vi "api_demo.vi"() -> ()   [LabVIEW 2017]
panel:
  in  "地址":string="127.0.0.1"
  in  "刷新":bool
  out "cz":dbl
  out "cy":dbl
  out "cx":dbl
  in  "LET":enum32{"回零", "扫描", "手动", "配置"}(tab)
  in  "组合框":string(combo)
  in  "去，并设置原点":bool
  in  "运行速度":dbl=50.0
  in  "去":bool
  in  "目标z":dbl
  in  "目标y":dbl=100.0
  in  "目标x":dbl=100.0
  in  "回零速度":dbl=20.0
  in  "回零":bool
  in  "slopey":dbl=100.0
  in  "slopex":dbl=100.0
  in  "ydir":bool=TRUE
  in  "xdir":bool=TRUE
  in  "scan v":dbl=50.0
  in  "退出扫描":bool
  in  "下一步":bool
  in  "开始":bool
  in  "type":string(combo)="zigzagx"
  out "状态":string
  in  "speed":dbl=50.0
  in  "step":dbl=50.0
  in  "Z-":bool
  in  "Z+":bool
  in  "Y+":bool
  in  "Y-":bool
  in  "X-":bool
  in  "X+":bool
  in  "复位":bool
  in  "刷新数值":bool
  in  "configrv":bool
  in  "configgap":bool
  in  "configwhz":bool
  in  "configdxdy":bool
  in  "configoxyz":bool
  in  "rv":dbl
  in  "zhome":dbl
  in  "gapspeed":dbl
  in  "gap":dbl
  in  "d":dbl
  in  "w":dbl
  in  "h":dbl
  in  "d2":dbl
  in  "d1":dbl
  in  "oz":dbl
  in  "oy":dbl
  in  "ox":dbl
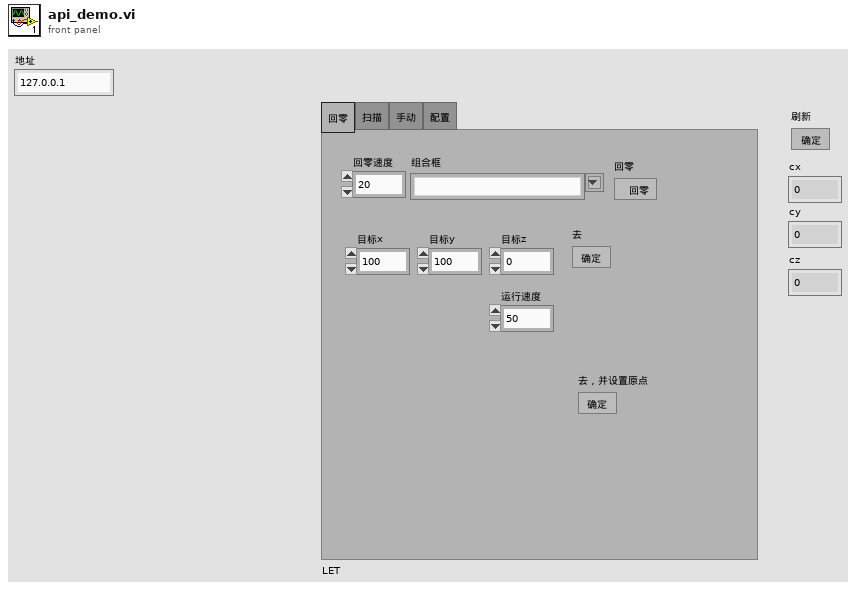
[diagram p1: front panel]
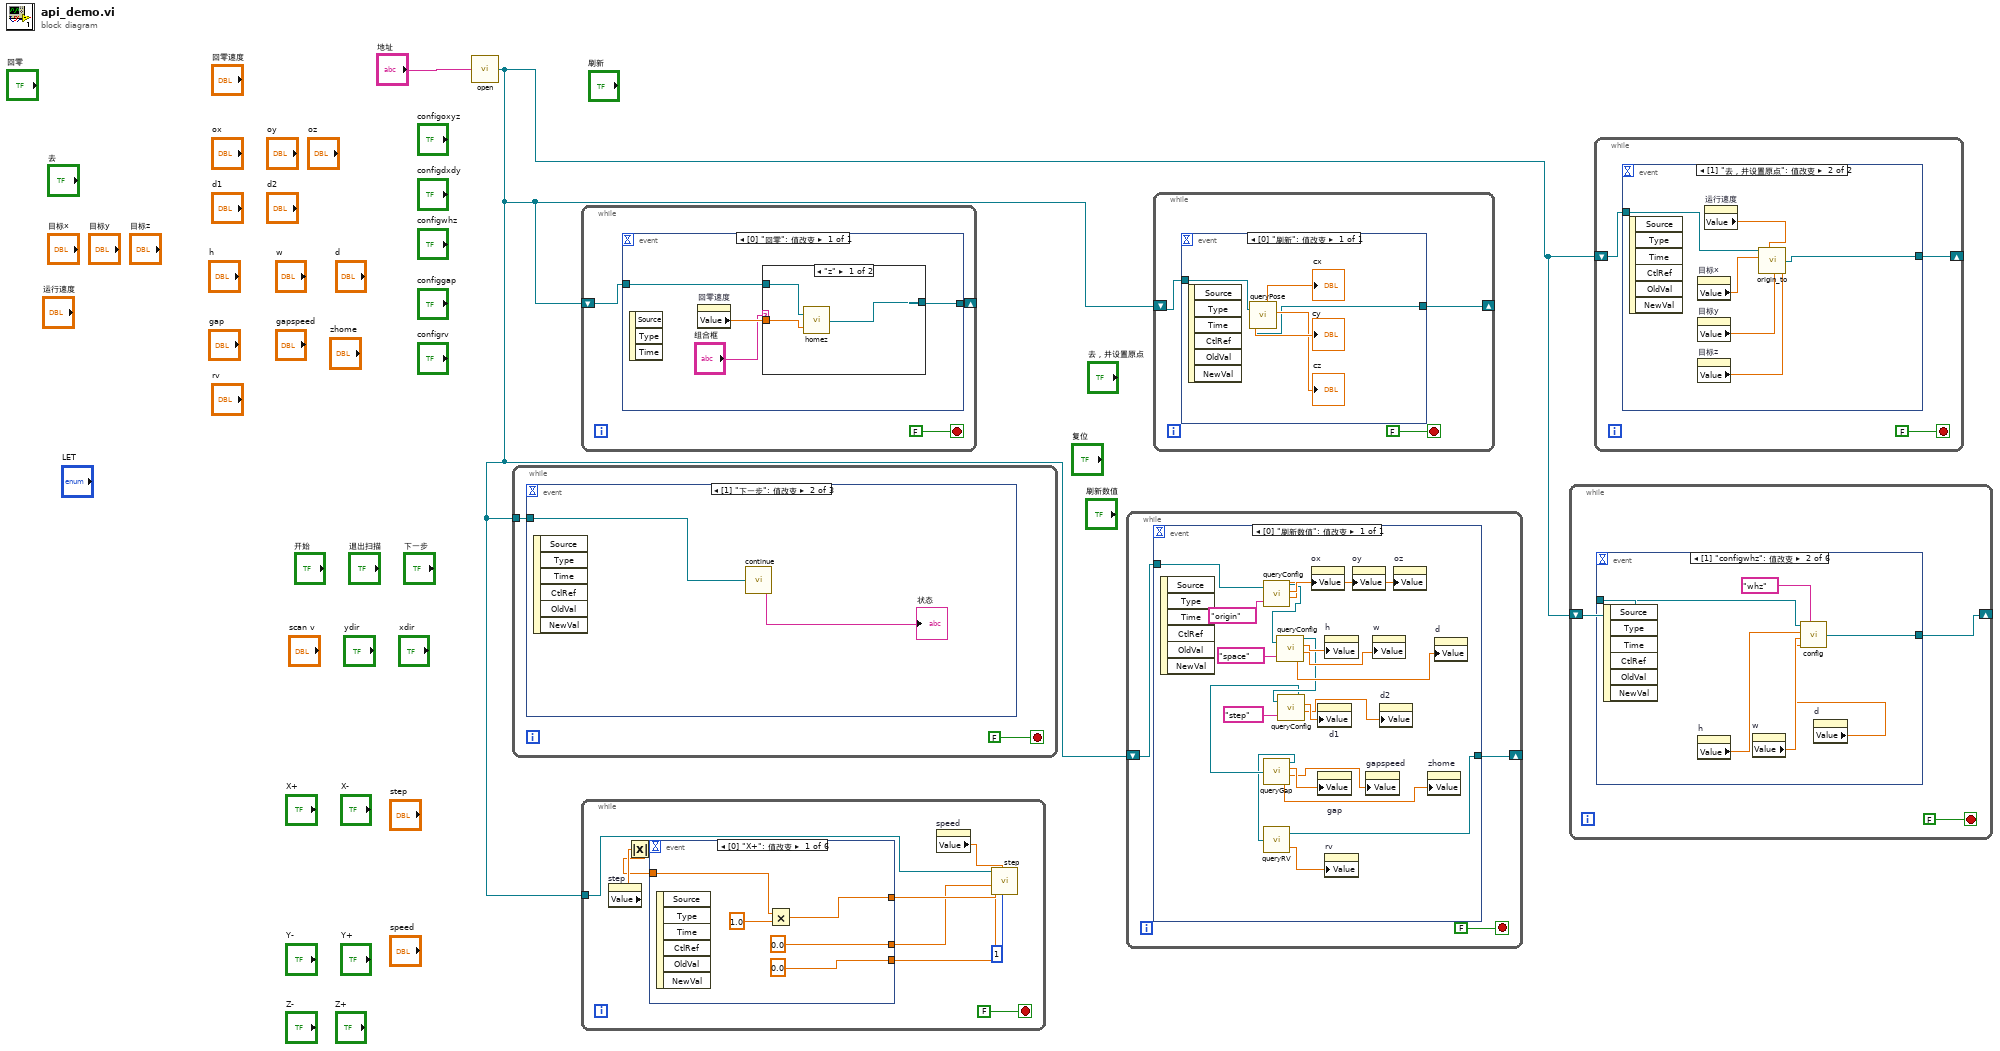
[diagram p0: block diagram]
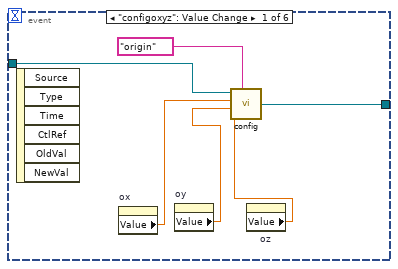
[diagram p2: hidden frame]
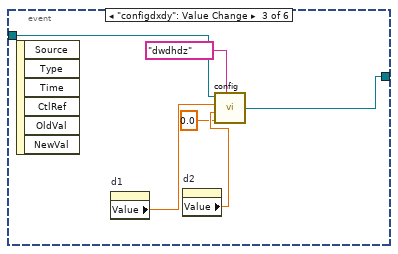
[diagram p3: hidden frame]
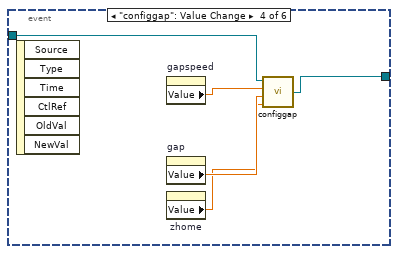
[diagram p4: hidden frame]
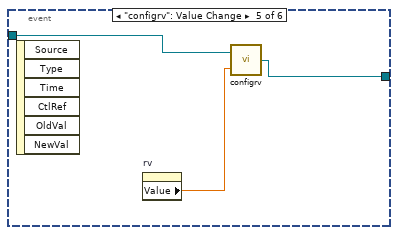
[diagram p5: hidden frame]
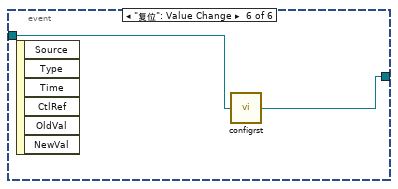
[diagram p6: hidden frame]
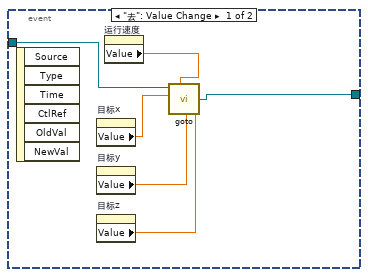
[diagram p7: hidden frame]
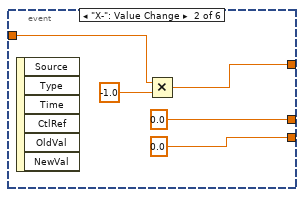
[diagram p8: hidden frame]
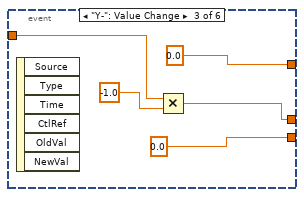
[diagram p9: hidden frame]
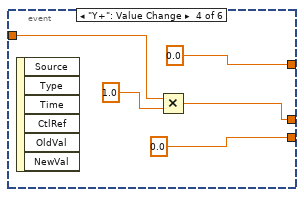
[diagram p10: hidden frame]
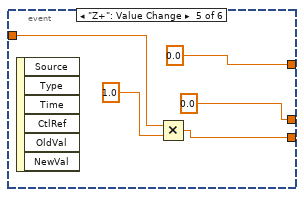
[diagram p11: hidden frame]
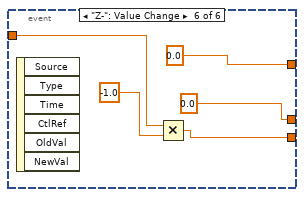
[diagram p12: hidden frame]
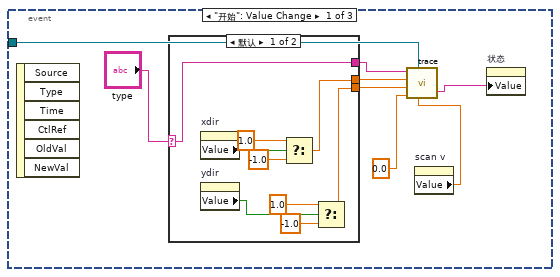
[diagram p13: hidden frame]
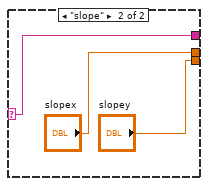
[diagram p14: hidden frame]
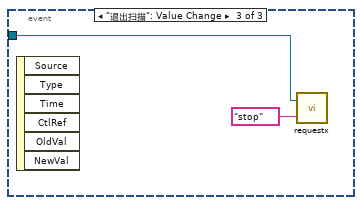
[diagram p15: hidden frame]
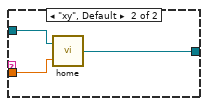
[diagram p16: hidden frame]
diagram:
  n1 = call "open.vi"("地址"="地址") -> ("连接ID"=w1:refnum<k5>)
  n2 = while {
    tunnel: w1 -> [w4]
    stop <- FALSE stop-if-true
    n3 = event shown="[1] \"下一步\": 值改变" {
      selector: _ -> [_ _ _]
      dyn-events: _ -> [_ _ _]
      timeout: _ -> [_ _ _]
      tunnel: w4 -> [w12 w26 w28]
      event "开始": Value Change {
        n4 = event-data() -> ()  [unwired: 1 in, 6 out]
        n5 = case shown="默认" "type" {
          selector: "type" -> [w13 w24]
          tunnel: [w18 "slopex"] -> w9
          tunnel: [w14 "slopey"] -> w8
          tunnel: [w13 w24] -> w5
          frame Default {
            n6 = property on="xdir" class="Bool (严格)"() -> ("Value"=w21:bool)  [unwired: 2 in, 2 out]
            n7 = property on="ydir" class="Bool (严格)"() -> ("Value"=w15:bool)  [unwired: 2 in, 2 out]
            n8 = Select(t=1.0, s=w21, f=-1.0) -> (s? t:f=w18:dbl)
            n9 = Select(t=1.0, s=w15, f=-1.0) -> (s? t:f=w14:dbl)
          }
          frame "slope" {
          }
        }
        n10 = property on="scan v" class="DigNum (严格)"() -> ("Value"=w10:dbl)  [unwired: 2 in, 2 out]
        n11 = call "trace.vi"("v"=w10, "连接ID"=w12, "z"=0.0, "y"=w8, "x"=w9, "type"=w5) -> ("输出状态"=w7:string)  [unwired: 1 out]
        n12 = property on="状态" class="Str"("Value"=w7) -> ()  [unwired: 2 in, 2 out]
      }
      event "下一步": Value Change {
        n13 = event-data() -> ()  [unwired: 1 in, 6 out]
        n14 = call "continue.vi"("连接ID"=w26) -> ("输出状态"=→"状态":string)  [unwired: 1 out]
      }
      event "退出扫描": Value Change {
        n15 = event-data() -> ()  [unwired: 1 in, 6 out]
        n16 = call "requestx.vi"("cmd"="stop", "连接ID"=w28) -> ()  [unwired: 1 out]
      }
    }
  }
  n17 = while {
    shift-right: [w30] -> _
    shift-left: w1 -> [w31]
    stop <- FALSE stop-if-true
    n18 = event shown="[0] \"回零\": 值改变" {
      selector: _ -> [_]
      dyn-events: _ -> [_]
      timeout: _ -> [_]
      tunnel: w31 -> [w35]
      tunnel: [w33] -> w30
      event "回零": Value Change {
        n19 = event-data() -> ()  [unwired: 1 in, 3 out]
        n20 = property on="回零速度" class="DigNum (严格)"() -> ("Value"=w34:dbl)  [unwired: 2 in, 2 out]
        n21 = case shown="\"z\"" "组合框" {
          tunnel: w35 -> [w38 w41]
          tunnel: w34 -> [w37 w40]
          tunnel: [w36 w39] -> w33
          frame "z" {
            n22 = call "homez.vi"("速度"=w37, "连接ID"=w38) -> ("连接ID"=w36:refnum<k5>)
          }
          frame "xy", Default {
            n23 = call "home.vi"("速度"=w40, "连接ID"=w41) -> ("连接ID"=w39:refnum<k5>)
          }
        }
      }
    }
  }
  n24 = while {
    tunnel: w1 -> [w50]
    stop <- FALSE stop-if-true
    n25 = property on="step" class="DigNum (严格)"() -> ("Value"=w48:dbl)  [unwired: 2 in, 2 out]
    n26 = Absolute Value(x=w48) -> (abs(x)=w47:dbl)
    n27 = event shown="[0] \"X+\": 值改变" {
      selector: _ -> [_ _ _ _ _ _]
      dyn-events: _ -> [_ _ _ _ _ _]
      timeout: _ -> [_ _ _ _ _ _]
      tunnel: w47 -> [w55 w60 w65 w70 w75 w80]
      tunnel: [w53 w58 0.0 ("y") 0.0 ("y") 0.0 ("y") 0.0 ("y")] -> w46
      tunnel: [0.0 ("y") 0.0 ("y") w62 w67 0.0 ("y") 0.0 ("y")] -> w45
      tunnel: [0.0 ("y") 0.0 ("y") 0.0 ("y") 0.0 ("y") w71 w76] -> w44
      event "X+": Value Change {
        n28 = event-data() -> ()  [unwired: 1 in, 6 out]
        n29 = Multiply(x=w55, y=1.0) -> (x*y=w53:dbl)
      }
      event "X-": Value Change {
        n30 = event-data() -> ()  [unwired: 1 in, 6 out]
        n31 = Multiply(x=w60, y=-1.0) -> (x*y=w58:dbl)
      }
      event "Y-": Value Change {
        n32 = event-data() -> ()  [unwired: 1 in, 6 out]
        n33 = Multiply(x=w65, y=-1.0) -> (x*y=w62:dbl)
      }
      event "Y+": Value Change {
        n34 = event-data() -> ()  [unwired: 1 in, 6 out]
        n35 = Multiply(x=w70, y=1.0) -> (x*y=w67:dbl)
      }
      event "Z+": Value Change {
        n36 = event-data() -> ()  [unwired: 1 in, 6 out]
        n37 = Multiply(x=w75, y=1.0) -> (x*y=w71:dbl)
      }
      event "Z-": Value Change {
        n38 = event-data() -> ()  [unwired: 1 in, 6 out]
        n39 = Multiply(x=w80, y=-1.0) -> (x*y=w76:dbl)
      }
    }
    n40 = property on="speed" class="DigNum (严格)"() -> ("Value"=w49:dbl)  [unwired: 2 in, 2 out]
    n41 = call "step.vi"("n"=1, "v"=w49, "z"=w44, "y"=w45, "x"=w46, "连接ID"=w50) -> ()  [unwired: 1 out]
  }
  n42 = while {
    shift-right: [w81] -> _
    shift-left: w1 -> [w83]
    stop <- FALSE stop-if-true
    n43 = event shown="[0] \"刷新数值\": 值改变" {
      selector: _ -> [_]
      dyn-events: _ -> [_]
      timeout: _ -> [_]
      tunnel: w83 -> [w104]
      tunnel: [w85] -> w81
      event "刷新数值": Value Change {
        n44 = event-data() -> ()  [unwired: 1 in, 6 out]
        n45 = call "queryConfig.vi"("连接ID"=w104, "item"="origin") -> ("连接ID输出"=w99:refnum<k5>, "x"=w102:dbl, "y"=w101:dbl, "z"=w100:dbl)
        n46 = call "queryConfig.vi"("连接ID"=w99, "item"="space") -> ("连接ID输出"=w94:refnum<k5>, "x"=w97:dbl, "y"=w96:dbl, "z"=w95:dbl)
        n47 = call "queryConfig.vi"("连接ID"=w94, "item"="step") -> ("连接ID输出"=w90:refnum<k5>, "x"=w92:dbl, "y"=w91:dbl)  [unwired: 1 out]
        n48 = call "queryGap.vi"("连接ID"=w90) -> ("连接ID输出"=w86:refnum<k5>, "gap"=w89:dbl, "gap speed"=w88:dbl, "z home speed"=w87:dbl)
        n49 = call "queryRV.vi"("连接ID"=w86) -> ("连接ID输出"=w85:refnum<k5>, "rv"=w84:dbl)
        n50 = property on="ox" class="DigNum (严格)"("Value"=w102) -> ()  [unwired: 2 in, 2 out]
        n51 = property on="d1" class="DigNum (严格)"("Value"=w92) -> ()  [unwired: 2 in, 2 out]
        n52 = property on="gap" class="DigNum (严格)"("Value"=w89) -> ()  [unwired: 2 in, 2 out]
        n53 = property on="h" class="DigNum (严格)"("Value"=w97) -> ()  [unwired: 2 in, 2 out]
        n54 = property on="rv" class="DigNum (严格)"("Value"=w84) -> ()  [unwired: 2 in, 2 out]
        n55 = property on="oy" class="DigNum (严格)"("Value"=w101) -> ()  [unwired: 2 in, 2 out]
        n56 = property on="gapspeed" class="DigNum (严格)"("Value"=w88) -> ()  [unwired: 2 in, 2 out]
        n57 = property on="w" class="DigNum (严格)"("Value"=w96) -> ()  [unwired: 2 in, 2 out]
        n58 = property on="d2" class="DigNum (严格)"("Value"=w91) -> ()  [unwired: 2 in, 2 out]
        n59 = property on="oz" class="DigNum (严格)"("Value"=w100) -> ()  [unwired: 2 in, 2 out]
        n60 = property on="zhome" class="DigNum (严格)"("Value"=w87) -> ()  [unwired: 2 in, 2 out]
        n61 = property on="d" class="DigNum (严格)"("Value"=w95) -> ()  [unwired: 2 in, 2 out]
      }
    }
  }
  n62 = while {
    shift-right: [w107] -> _
    shift-left: w1 -> [w106]
    stop <- FALSE stop-if-true
    n63 = event shown="[0] \"刷新\": 值改变" {
      selector: _ -> [_]
      dyn-events: _ -> [_]
      timeout: _ -> [_]
      tunnel: [w109] -> w107
      tunnel: w106 -> [w108]
      event "刷新": Value Change {
        n64 = event-data() -> ()  [unwired: 1 in, 6 out]
        n65 = call "queryPose.vi"("连接ID"=w108) -> ("连接ID输出"=w109:refnum<k5>, "x"=→"cx":dbl, "y"=→"cy":dbl, "z"=→"cz":dbl)  [unwired: 3 out]
      }
    }
  }
  n66 = while {
    shift-right: [w113] -> _
    shift-left: w1 -> [w114]
    stop <- FALSE stop-if-true
    n67 = event shown="[1] \"configwhz\": 值改变" {
      selector: _ -> [_ _ _ _ _ _]
      dyn-events: _ -> [_ _ _ _ _ _]
      timeout: _ -> [_ _ _ _ _ _]
      tunnel: w114 -> [w120 w123 w133 w138 w141 w143]
      tunnel: [w119 w124 w132 w137 w139 w142] -> w113
      event "configoxyz": Value Change {
        n68 = event-data() -> ()  [unwired: 1 in, 6 out]
        n69 = property on="ox" class="DigNum (严格)"() -> ("Value"=w118:dbl)  [unwired: 2 in, 2 out]
        n70 = property on="oy" class="DigNum (严格)"() -> ("Value"=w117:dbl)  [unwired: 2 in, 2 out]
        n71 = property on="oz" class="DigNum (严格)"() -> ("Value"=w116:dbl)  [unwired: 2 in, 2 out]
        n72 = call "config.vi"("连接ID"=w120, "x"=w118, "y"=w117, "z"=w116, "item"="origin") -> ("连接ID输出"=w119:refnum<k5>)
      }
      event "configwhz": Value Change {
        n73 = event-data() -> ()  [unwired: 1 in, 6 out]
        n74 = property on="h" class="DigNum (严格)"() -> ("Value"=w127:dbl)  [unwired: 2 in, 2 out]
        n75 = property on="w" class="DigNum (严格)"() -> ("Value"=w126:dbl)  [unwired: 2 in, 2 out]
        n76 = property on="d" class="DigNum (严格)"() -> ("Value"=w125:dbl)  [unwired: 2 in, 2 out]
        n77 = call "config.vi"("连接ID"=w123, "x"=w127, "y"=w126, "z"=w125, "item"="whz") -> ("连接ID输出"=w124:refnum<k5>)
      }
      event "configdxdy": Value Change {
        n78 = event-data() -> ()  [unwired: 1 in, 6 out]
        n79 = property on="d1" class="DigNum (严格)"() -> ("Value"=w130:dbl)  [unwired: 2 in, 2 out]
        n80 = property on="d2" class="DigNum (严格)"() -> ("Value"=w129:dbl)  [unwired: 2 in, 2 out]
        n81 = call "config.vi"("连接ID"=w133, "x"=w130, "y"=w129, "z"=0.0, "item"="dwdhdz") -> ("连接ID输出"=w132:refnum<k5>)
      }
      event "configgap": Value Change {
        n82 = event-data() -> ()  [unwired: 1 in, 6 out]
        n83 = property on="gapspeed" class="DigNum (严格)"() -> ("Value"=w136:dbl)  [unwired: 2 in, 2 out]
        n84 = property on="gap" class="DigNum (严格)"() -> ("Value"=w135:dbl)  [unwired: 2 in, 2 out]
        n85 = property on="zhome" class="DigNum (严格)"() -> ("Value"=w134:dbl)  [unwired: 2 in, 2 out]
        n86 = call "configgap.vi"("zhomespeed"=w134, "gap"=w135, "gapspeed"=w136, "连接ID"=w138) -> ("连接ID输出"=w137:refnum<k5>)
      }
      event "configrv": Value Change {
        n87 = event-data() -> ()  [unwired: 1 in, 6 out]
        n88 = property on="rv" class="DigNum (严格)"() -> ("Value"=w140:dbl)  [unwired: 2 in, 2 out]
        n89 = call "configrv.vi"("rv"=w140, "连接ID"=w141) -> ("连接ID输出"=w139:refnum<k5>)
      }
      event "复位": Value Change {
        n90 = event-data() -> ()  [unwired: 1 in, 6 out]
        n91 = call "configrst.vi"("连接ID"=w143) -> ("连接ID输出"=w142:refnum<k5>)
      }
    }
  }
  n92 = while {
    shift-right: [w145] -> _
    shift-left: w1 -> [w146]
    stop <- FALSE stop-if-true
    n93 = event shown="[1] \"去，并设置原点\": 值改变" {
      selector: _ -> [_ _]
      dyn-events: _ -> [_ _]
      timeout: _ -> [_ _]
      tunnel: w146 -> [w152 w158]
      tunnel: [w147 w153] -> w145
      event "去": Value Change {
        n94 = event-data() -> ()  [unwired: 1 in, 6 out]
        n95 = property on="目标x" class="DigNum (严格)"() -> ("Value"=w150:dbl)  [unwired: 2 in, 2 out]
        n96 = property on="目标y" class="DigNum (严格)"() -> ("Value"=w149:dbl)  [unwired: 2 in, 2 out]
        n97 = property on="目标z" class="DigNum (严格)"() -> ("Value"=w148:dbl)  [unwired: 2 in, 2 out]
        n98 = property on="运行速度" class="DigNum (严格)"() -> ("Value"=w151:dbl)  [unwired: 2 in, 2 out]
        n99 = call "goto.vi"("连接ID"=w152, "x"=w150, "y"=w149, "z"=w148, "v"=w151) -> ("连接ID"=w147:refnum<k5>)
      }
      event "去，并设置原点": Value Change {
        n100 = event-data() -> ()  [unwired: 1 in, 6 out]
        n101 = property on="目标x" class="DigNum (严格)"() -> ("Value"=w156:dbl)  [unwired: 2 in, 2 out]
        n102 = property on="目标y" class="DigNum (严格)"() -> ("Value"=w155:dbl)  [unwired: 2 in, 2 out]
        n103 = property on="目标z" class="DigNum (严格)"() -> ("Value"=w154:dbl)  [unwired: 2 in, 2 out]
        n104 = property on="运行速度" class="DigNum (严格)"() -> ("Value"=w157:dbl)  [unwired: 2 in, 2 out]
        n105 = call "origin_to.vi"("连接ID"=w158, "x"=w156, "y"=w155, "z"=w154, "v"=w157) -> ("连接ID输出"=w153:refnum<k5>)
      }
    }
  }
